vi "List ID.vi"(7 "Parent ID":string, 8 "Error In":errorcluster, 11 "Tree Manager":T1) -> (0 "Error Out":errorcluster, 1 "Child IDs":string[](array[string]), 2 "Child Names":string[](array[string]), 3 "Tree Manager":T1)   [LabVIEW 2016, in "Tree Manager.lvclass"]
doc: "List the direct Children of the wired in Parent Tree. If the Parent ID input is left unwired all Trees ID are listed.\n\nThe list order is random."
uses:
  Tree Manager.lvclass
  Typedefs/Session Handle.ctl
  Tree Manager.lvclass/Tree Manager.ctl
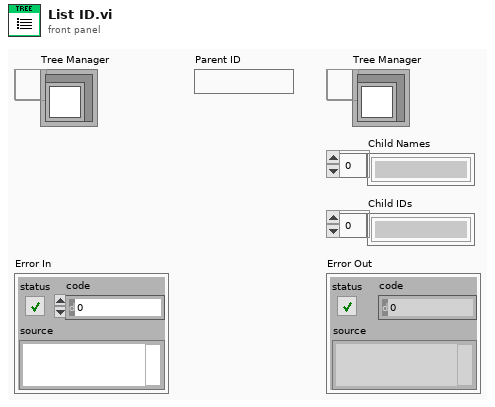
[diagram p1: front panel]
types:
  T1 = typedef "Tree Manager.lvclass/Session Handle.ctl" = refnum<data-value>
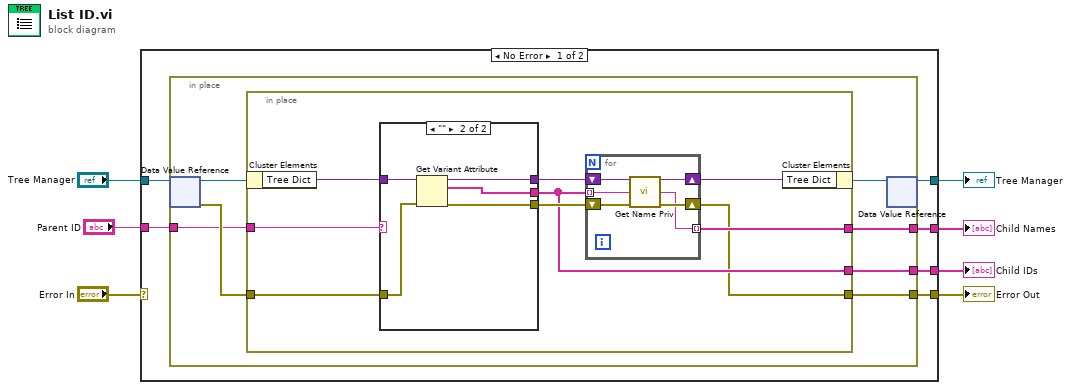
[diagram p0: block diagram]
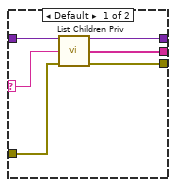
[diagram p2: hidden frame]
diagram:
  n1 = case shown="No Error" "Error In" {
    selector: "Error In" -> [_ w47]
    tunnel: "Tree Manager" -> [w13 w48]
    tunnel: [w12 w48] -> w6
    tunnel: [w11 w47] -> w4
    tunnel: "Parent ID" -> [w10 _]
    tunnel: [w9 _] -> w2
    tunnel: [w8 _] -> w1
    frame No Error {
      n2 = in-place {
        in-place-border: [w19] -> w11
        in-place-border: w10 -> [w16]
        in-place-border: [w15] -> w9
        in-place-border: [w14] -> w8
        n3 = in-place-dvr #1(w13) -> (w20:refnum<class "Tree Manager.lvclass">, w17:errorcluster)
        n4 = in-place {
          in-place-border: [w22] -> w19
          in-place-border: w17 -> [w28]
          in-place-border: w16 -> [w27]
          in-place-border: [w24] -> w15
          in-place-border: [w23] -> w14
          n5 = in-place-cluster #2(w20) -> ("Tree Dict"=w29:variant)
          n6 = case shown="\"\"" w27 {
            selector: w27 -> [w40 _]
            tunnel: w29 -> [w41 w46]
            tunnel: [w37 w45] -> w26
            tunnel: w28 -> [w39 w44]
            tunnel: [w36 w43] -> w25
            tunnel: [w38 w42] -> w24
            frame Default {
              n7 = call "List Children Priv.vi"("Tree Dictionary"=w41, "Parent ID"=w40, "Error In"=w39) -> ("Tree Dictionary Out"=w37:variant, "Child IDs"=w38:string[], "Error Out"=w36:errorcluster)  [unwired: 10 in]
            }
            frame "" {
              n8 = Get Variant Attribute(Variant=w46, error in=w44) -> (duplicate Variant=w45:variant, names=w42:string[], error out=w43:errorcluster)  [unwired: 2 in, 1 out]
            }
          }
          n9 = for {
            shift-right: [w34] -> w21
            shift-left: w26 -> [w35]
            tunnel: w24 -> [w32] mode=indexing
            shift-right: [w31] -> w22
            shift-left: w25 -> [w33]
            tunnel: [w30] -> w23 mode=indexing
            n10 = call "Get Name Priv.vi"("Tree Dictionary"=w35, "Unique ID"=w32, "error in"=w33) -> ("Tree Dictionary Out"=w34:variant, "Name"=w30:string, "error out"=w31:errorcluster)  [unwired: 10 in]
          }
          n11 = in-place-cluster #2("Tree Dict"=w21) -> (w18:refnum<class "Tree Manager.lvclass">)
        }
        n12 = in-place-dvr #1(w18) -> (w12:T1)  [unwired: 1 out]
      }
    }
    frame Error {
    }
  }
  "Tree Manager" <- w6
  "Error Out" <- w4
  "Child IDs" <- w2
  "Child Names" <- w1
